vi "Render to Writer.vi"(7 "Data":cluster{"Key":string, "Value":variant}[](array[cluster]), 8 "Error In":errorcluster, 10 "Writer In":refnum<class "Abstract.lvclass">, 11 "Render In":refnum<class "Render.lvclass">) -> (0 "Error Out":errorcluster, 2 "Writer Out":refnum<class "Abstract.lvclass">, 3 "Render Out":refnum<class "Render.lvclass">)   [LabVIEW 2018, in "Toolkit.lvlib" / "Render.lvclass"]
uses:
  Render.lvclass
  Writers/Abstract/Abstract.lvclass
  Render.lvclass/Render.ctl
  Nodes/Root/Root.lvclass
  Nodes/Abstract/Abstract.lvclass
  Compiler/Compiler.lvclass
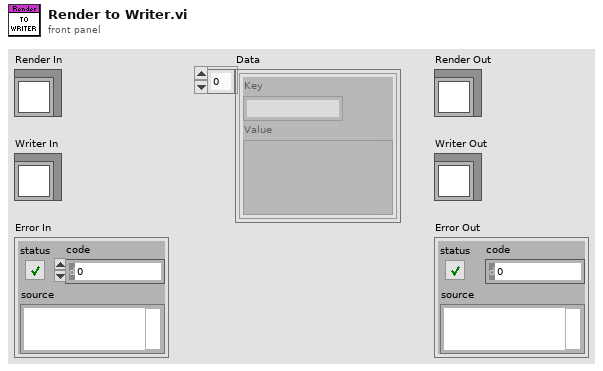
[diagram p1: front panel]
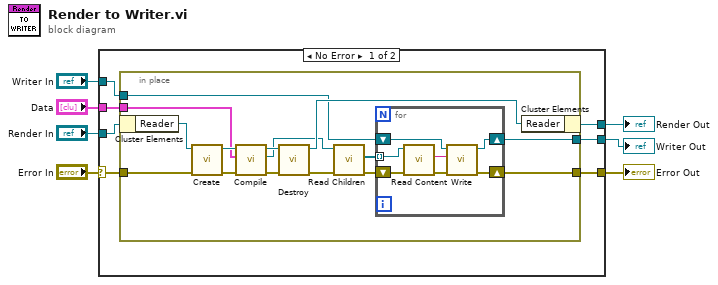
[diagram p0: block diagram]
diagram:
  n1 = case shown="No Error" "Error In" {
    selector: "Error In" -> [w13 w37]
    tunnel: "Render In" -> [w14 w38]
    tunnel: [w12 w38] -> w5
    tunnel: [w9 w37] -> w4
    tunnel: "Data" -> [w11 _]
    tunnel: "Writer In" -> [w10 _]
    tunnel: [w8 _] -> w1
    frame No Error {
      n2 = in-place {
        in-place-border: w13 -> [w28]
        in-place-border: w11 -> [w22]
        in-place-border: w10 -> [w16]
        in-place-border: [w17] -> w9
        in-place-border: [w15] -> w8
        n3 = in-place-cluster #1(w14) -> ("Reader"=w29:refnum<class "Abstract.lvclass">)
        n4 = call "Create.vi"("Error In"=w28, "Reader"=w29) -> ("Error Out"=w26:errorcluster, "Compiler"=w27:refnum<class "Compiler.lvclass">)  [unwired: 8 in]
        n5 = call "Compile.vi"("Error In"=w26, "Data"=w22, "Compiler In"=w27) -> ("Error Out"=w24:errorcluster, "Abstract Syntax Tree"=w21:refnum<class "Root.lvclass">, "Compiler Out"=w25:refnum<class "Compiler.lvclass">)  [unwired: 6 in]
        n6 = call "Destroy.vi"("Error In"=w24, "Compiler"=w25) -> ("Error Out"=w20:errorcluster, "Reader"=w23:refnum<class "Abstract.lvclass">)  [unwired: 8 in]
        n7 = call-dynamic "Read Children.vi"("Error In"=w20, "NonTerminal In"=w21) -> ("Error Out"=w18:errorcluster, "Children"=w19:refnum<class "Abstract.lvclass">[])  [unwired: 7 in, 1 out]
        n8 = for {
          tunnel: w19 -> [w33] mode=indexing
          shift-right: [w36] -> w17
          shift-left: w18 -> [w32]
          shift-right: [w34] -> w15
          shift-left: w16 -> [w35]
          n9 = call-dynamic "Read Content.vi"("Error In"=w32, "Abstract In"=w33) -> ("Error Out"=w30:errorcluster, "Content"=w31:string)  [unwired: 7 in, 1 out]
          n10 = call-dynamic "Write.vi"("Error In"=w30, "Content"=w31, "Writer In"=w35) -> ("Error Out"=w36:errorcluster, "Writer Out"=w34:refnum<class "Abstract.lvclass">)  [unwired: 7 in]
        }
        n11 = in-place-cluster #1("Reader"=w23) -> (w12:refnum<class "Render.lvclass">)
      }
    }
    frame Error {
    }
  }
  "Render Out" <- w5
  "Error Out" <- w4
  "Writer Out" <- w1
